vi "method2.vi"(8 "error in (no error)":errorcluster, 10 "RefNum":i32, 11 "ContentClass in":refnum<class "ContentClass.lvclass">) -> (0 "error out":errorcluster, 2 "Boolean":bool, 3 "ContentClass out":refnum<class "ContentClass.lvclass">)   [LabVIEW 2019, in "lv-providershell-example3.lvlib" / "ContentClass.lvclass"]
uses:
  ContentClass.lvclass
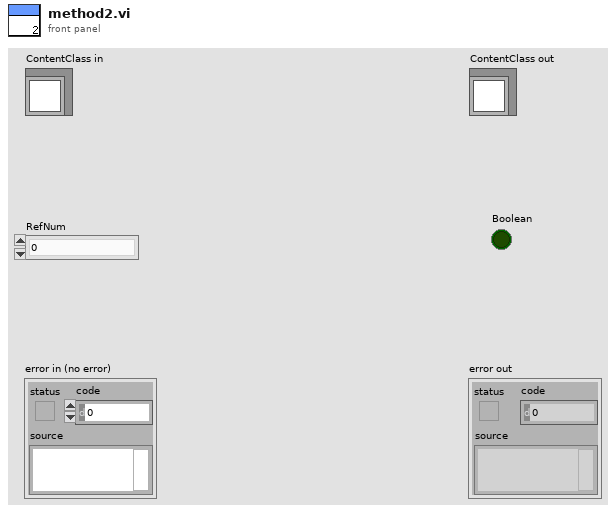
[diagram p1: front panel]
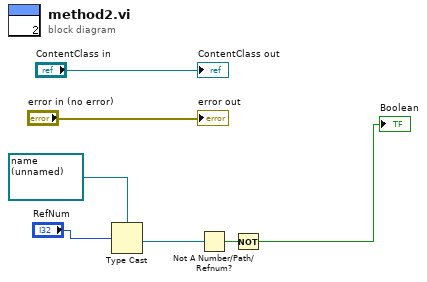
[diagram p0: block diagram]
diagram:
  n1 = Type Cast(type=refnum<queue> refnum ("queue out"), x="RefNum") -> (*(type *) &x=w2:refnum<queue>)
  n2 = Not A Number/Path/Refnum?(number/path/refnum=w2) -> (NaN/Path/Refnum?=w5:bool)
  n3 = Not(x=w5) -> (.not. x?=→"Boolean":bool)
  "error out" <- "error in (no error)"
  "ContentClass out" <- "ContentClass in"
